vi "KH7008 Set All.vi"(0 "Channel":u16(ring)=1 items=["Channel 1"=1, "Channel 2"=2, "Channel 3"=3, "Channel 4"=4, "Channel 5"=5, "Channel 6"=6, "Channel 7"=7, "Channel 8"=8], 1 "VISA Refnum in":refnum<visa-resource-name>="COM1", 2 "Coupling":u16(ring)=2 items=["AC"=1, "DC"=2], 3 "Shunt Resistor":u16(ring)=1 items=["Open"=1, "50 Ohms"=2, "500 Ohms"=3, "5k Ohms"=4, "50k Ohms"=5], 4 "Input Coupling":u16(ring)=3 items=["Off (both off)"=1, "SE + (- grounded)"=2, "SE - (+ grounded)"=3, "Diff (both on)"=4], 5 "Gain":u16(ring)=1 items=["1x"=1, "10x"=2, "100x"=3, "1000x"=4], 7 "Bandwidth Filter":u16(ring)=2 items=["OFF"=1, "ON"=2], 8 "error in (no error)":errorcluster) -> (9 "error out":errorcluster)   [LabVIEW 2013]
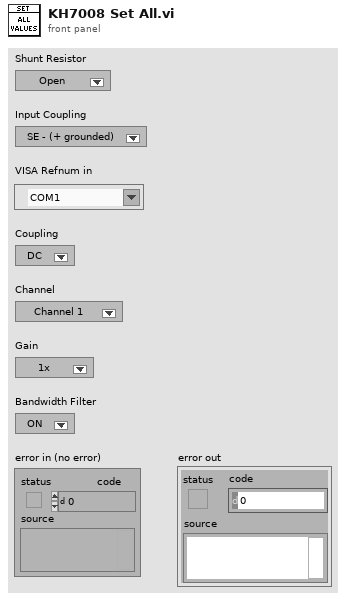
[diagram p1: front panel]
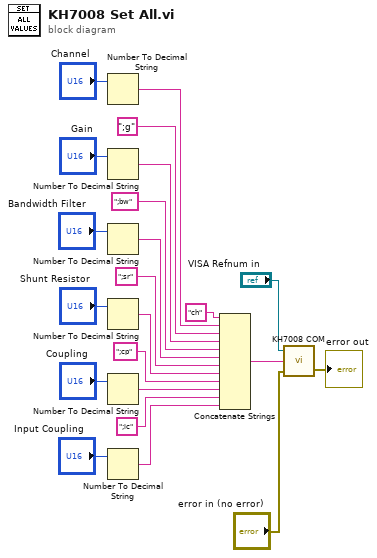
[diagram p0: block diagram]
diagram:
  n1 = Number To Decimal String(number="Channel") -> (decimal integer string=w19:string)  [unwired: 1 in]
  n2 = Number To Decimal String(number="Gain") -> (decimal integer string=w21:string)  [unwired: 1 in]
  n3 = Number To Decimal String(number="Bandwidth Filter") -> (decimal integer string=w4:string)  [unwired: 1 in]
  n4 = Number To Decimal String(number="Shunt Resistor") -> (decimal integer string=w5:string)  [unwired: 1 in]
  n5 = Number To Decimal String(number="Coupling") -> (decimal integer string=w6:string)  [unwired: 1 in]
  n6 = Number To Decimal String(number="Input Coupling") -> (decimal integer string=w7:string)  [unwired: 1 in]
  n7 = Concatenate Strings("ch" ("string"), w19, ";g" ("string"), w21, ";bw" ("string"), w4, ";sr" ("string"), w5, ";cp" ("string"), w6, ";ic" ("string"), w7) -> (w22:string)
  n8 = call "KH7008 COM.vi"("error in (no error)"="error in (no error)", "Command"=w22, "VISA Refnum in"="VISA Refnum in") -> ("error out"=→"error out":errorcluster)  [unwired: 1 out]
